vi "Trigger_Delay.vi"() -> ()   [LabVIEW 2011]
doc: "I. Description:\nThis example demonstrates how to continuously output a waveform using an internal sample clock. The automatic regeneration of data has been disabled, so new data has to be provided throughout the duration of the continuous Analog Output operation. This allows the generation of any arbitrary frequency as this VI computes new data for each iteration of the loop, maintaining phase continuity of the signal.\n\nII. Instructions for Running:\n1. Select the Physical Channel to correspond to where your signal is output on the DAQ device.\n2. Enter the Minimum and Maximum Voltage range.\n3. Specify the desired Sample Clock Rate of the output Waveform. Higher sample clock rates will produce a smoother waveform.\n4. Manually specify the Analog Output buffer size, in number of samples. A larger buffer would help non-regenerative operations avoid errors due to occasional high CPU load. \nNote: \nThe Analog Output buffer has to be at least as big as the amount of data being written to the board per iteration. The recommended buffer size would be at least twice the amount of data being written to the board per iteration.\n5. Enter the Waveform Information. See the documentation of the Basic Function Generator SubVI for information on each parameter.\n\nIII. Block Diagram Steps:\n1. Create an Analog Output Voltage channel.\n2. Configure the task to prohibit the automatic regeneration of data.\n3. Call the DAQmx (Sample Clock) VI to set the sample clock rate. Additionally, set the sample mode to Continuous.\n4. Read the actual sample clock rate (eventually coerced depending on the hardware used). \n5. Compute the desired waveform, using the buffer size and the actual update rate. This VI keeps track of the phase of the waveform to ensure that the generated signal is continuous.\n6. Write the waveform to the output buffer. \n7a. Call the Start VI. This is only needed when the loop is executed for the first time.\n7b. Do nothing.\n8. Loop continuously until user presses the Stop button. Every iteration computes and writes a new waveform to the buffer.\n9. Call the Clear Task VI to clear the Task.\n10. Use the popup dialog box to display an error or warning if any.\n\nIV. I/O Connections Overview:\nMake sure your signal output terminal matches the Physical Channel I/O Control. For further connection information, refer to your hardware reference manual."
uses:
  <vilib>/Utility/error.llb/DialogType.ctl
  <vilib>/DAQmx/write.llb/DAQmx Write (Analog 1D DBL 1Chan NSamp).vi
  <vilib>/DAQmx/read.llb/DAQmx Read (Analog Wfm 1Chan NSamp).vi
  <vilib>/DAQmx/write.llb/DAQmx Write (Analog Wfm 1Chan NSamp).vi
  <vilib>/DAQmx/create/channels.llb/DAQmx Create Channel (AI-Voltage-Basic).vi
  <vilib>/DAQmx/configure/timing.llb/DAQmx Timing (Sample Clock).vi
  <vilib>/DAQmx/create/channels.llb/DAQmx Create Channel (AO-Voltage-Basic).vi
  <vilib>/DAQmx/miscellaneous.llb/DAQmx Fill In Error Info.vi
  Program Files/National Instruments/LabVIEW 2011/resource/objmgr/daqmx.rc
panel:
  in  "AI Physical Channels":tag="Dev1/ai0"
  in  "Delay Between \nAI and AO (seconds)":dbl=0.25 format="%0.2f"
  in  "Sample Clock Rate (Hz)":dbl=100.0 format="%0.2f"
  in  "Minimum Value":dbl=-5.0 format="%0.2f"
  in  "Maximum Value":dbl=5.0 format="%0.2f"
  in  "stop":bool
  # "Channel Parameters"
  # "Timing Parameters"
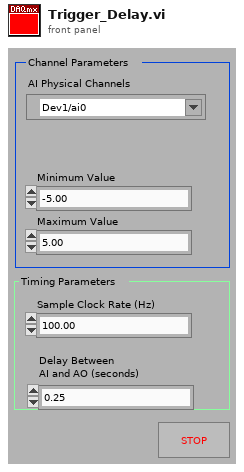
[diagram p1: front panel]
types:
  T1 = typedef "DialogType.ctl" = u16
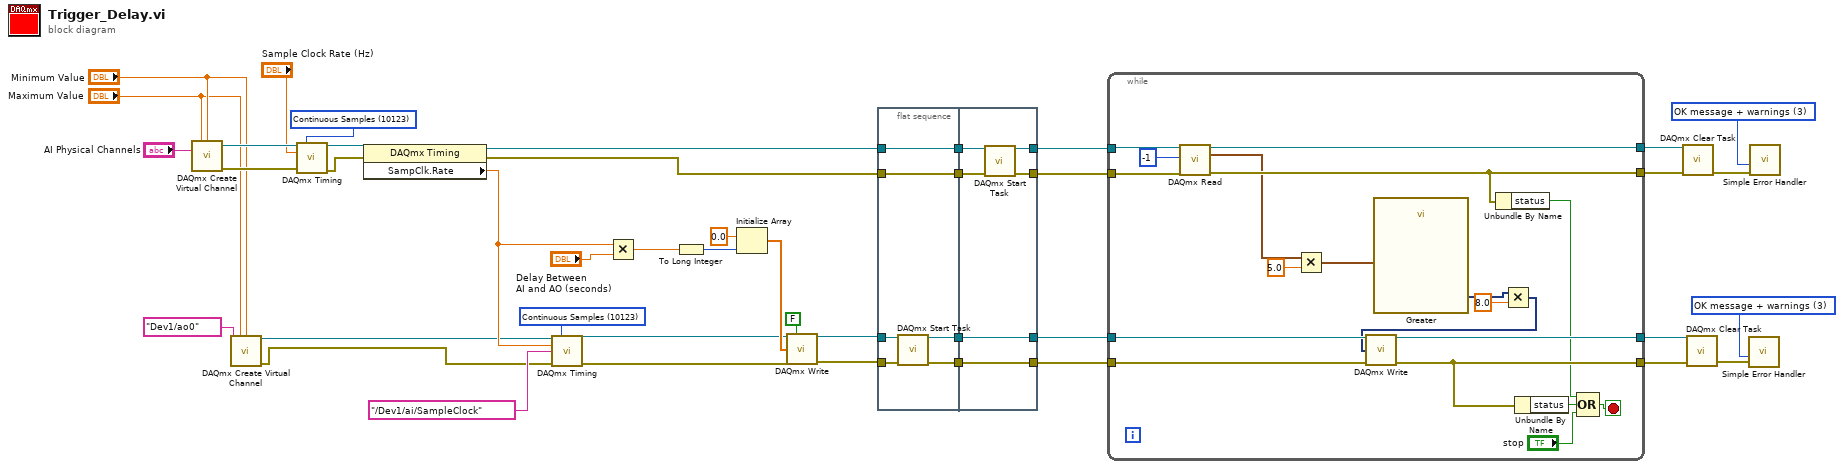
[diagram p0: block diagram]
diagram:
  w12 = T1 3 items=["no dialog", "OK message", "continue or stop message", "OK message + warnings", "continue/stop + warnings"] ("type of dialog (OK msg:1)")
  w38 = 10123 items=["Finite Samples"=10178, "Continuous Samples"=10123] ("sample mode")
  w41 = T1 3 items=["no dialog", "OK message", "continue or stop message", "OK message + warnings", "continue/stop + warnings"] ("type of dialog (OK msg:1)")
  w42 = 10123 items=["Finite Samples"=10178, "Continuous Samples"=10123] ("sample mode")
  n1 = call-poly <vilib>:"DAQmx Create Virtual Channel.vi"("maximum value"="Maximum Value", "minimum value"="Minimum Value", "physical channels"="AI Physical Channels") -> ("task out"=w39:refnum<k21>, "error out"=w40:errorcluster)  [unwired: 6 in, 5 out]
  n2 = call-poly <vilib>:"DAQmx Create Virtual Channel.vi"("maximum value"="Maximum Value", "minimum value"="Minimum Value", "physical channels"=tag "Dev1/ao0") -> ("task out"=w2:refnum<k21>, "error out"=w3:errorcluster)  [unwired: 6 in, 5 out]
  n3 = call-poly <vilib>:"DAQmx Timing.vi"("task/channels in"=w39, "sample mode"=w38, "rate"="Sample Clock Rate (Hz)", "error in"=w40) -> ("task out"=w20:refnum<k21>, "error out"=w21:errorcluster)  [unwired: 3 in, 7 out]
  n4 = property class="DAQmx Timing"(reference=w20, error in=w21) -> (reference out=w7:refnum<k21>, error out=w8:errorcluster, "SampClk.Rate"=w18:dbl)
  n5 = call-poly <vilib>:"DAQmx Timing.vi"("task/channels in"=w2, "sample mode"=w42, "rate"=w18, "source"=tag "/Dev1/ai/SampleClock", "error in"=w3) -> ("task out"=w4:refnum<k21>, "error out"=w5:errorcluster)  [unwired: 2 in, 7 out]
  n6 = Multiply(x=w18, y="Delay Between \nAI and AO (seconds)") -> (x*y=w17:dbl)
  n7 = To Long Integer(number=w17) -> (32bit integer=w25:i32)
  n8 = Initialize Array(0.0 ("element"), w25) -> (w23:dbl[])
  n9 = call-poly <vilib>:"DAQmx Write.vi"("task/channels in"=w4, "auto start"=FALSE, "data"=w23, "error in"=w5) -> ("task out"=w34:refnum<k21>, "error out"=w33:errorcluster)  [unwired: 10 out]
  n10 = flat-sequence {
    tunnel: [w49] -> w37
    tunnel: w8 -> [w49]
    tunnel: w34 -> [w48]
    tunnel: w33 -> [w47]
    tunnel: [w46] -> w36
    tunnel: [w45] -> w35
    tunnel: [w44] -> w32
    tunnel: w7 -> [w44]
    tunnel: w37 -> [w55]
    tunnel: [w54] -> w30
    tunnel: [w53] -> w29
    tunnel: w36 -> [w53]
    tunnel: [w52] -> w28
    tunnel: w35 -> [w52]
    tunnel: w32 -> [w51]
    tunnel: [w50] -> w31
    frame #0 {
      n11 = call <vilib>:"DAQmx Start Task.vi"("task/channels in"=w48, "error in"=w47) -> ("task out"=w46:refnum<k21>, "error out"=w45:errorcluster)  [unwired: 12 out]
    }
    frame #1 {
      n12 = call <vilib>:"DAQmx Start Task.vi"("task/channels in"=w51, "error in"=w55) -> ("task out"=w50:refnum<k21>, "error out"=w54:errorcluster)  [unwired: 12 out]
    }
  }
  n13 = while {
    tunnel: w31 -> [w68]
    tunnel: w30 -> [w67]
    tunnel: w29 -> [w70]
    tunnel: w28 -> [w71]
    tunnel: [w69] -> w27
    tunnel: [w66] -> w14
    tunnel: [w63] -> w15
    tunnel: [w64] -> w16
    stop <- w74 stop-if-true
    n14 = call-poly <vilib>:"DAQmx Read.vi"("task/channels in"=w68, "number of samples per channel"=-1, "error in"=w67) -> ("task out"=w66:refnum<k21>, "data"=w61:waveform(dbl), "error out"=w63:errorcluster)  [unwired: 10 out]
    n15 = Multiply(x=w61, y=5.0) -> (x*y=w59:waveform(dbl))
    n16 = call "Greater"("Operand 1"=w59) -> ("Result"=w58:dynamicdata)  [unwired: 9 in, 1 out]
    n17 = Unbundle By Name(w63) -> ("status"=w62:bool)
    n18 = Multiply(x=w58, y=8.0) -> (x*y=w56:dynamicdata)
    n19 = call-poly <vilib>:"DAQmx Write.vi"("task/channels in"=w70, "data"=w56, "error in"=w71) -> ("task out"=w64:refnum<k21>, "error out"=w69:errorcluster)  [unwired: 1 in, 10 out]
    n20 = Unbundle By Name(w69) -> ("status"=w73:bool)
    n21 = Compound Arithmetic op=OR(w62, w73, "stop") -> (w74:bool)
  }
  n22 = call <vilib>:"DAQmx Clear Task.vi"("task in"=w14, "error in"=w15) -> ("error out"=w13:errorcluster)  [unwired: 13 out]
  n23 = call <vilib>:"DAQmx Clear Task.vi"("task in"=w16, "error in"=w27) -> ("error out"=w43:errorcluster)  [unwired: 13 out]
  n24 = call <vilib>:"Simple Error Handler.vi"("type of dialog (OK msg:1)"=w41, "error in (no error)"=w43) -> ()  [unwired: 8 out]
  n25 = call <vilib>:"Simple Error Handler.vi"("type of dialog (OK msg:1)"=w12, "error in (no error)"=w13) -> ()  [unwired: 8 out]
